vi "1553B-PACKET-2.vi"(0 "数组输入":u8[](array[numeric])) -> (1 "东向加速度":i32, 2 "地向力加速度":i32, 3 "传感器信号":cluster{"陀螺温度":i16, "加计温度":i16}, 4 "俯仰角速率":i16, 6 "北向加速度":i32, 8 "滚转角速率":i16, 10 "航向角速率":i16, 12 "法向过载":i16, 13 "轴向过载":i16, 14 "侧向过载":i16, 15 "地向速度":i32)   [LabVIEW 2012]
uses:
  index-i16.vi
  XX-I16.vi
  index-i32.vi
  XX-I32.vi
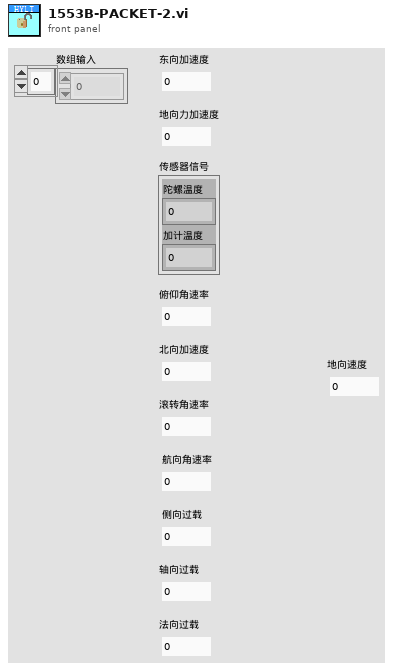
[diagram p1: front panel]
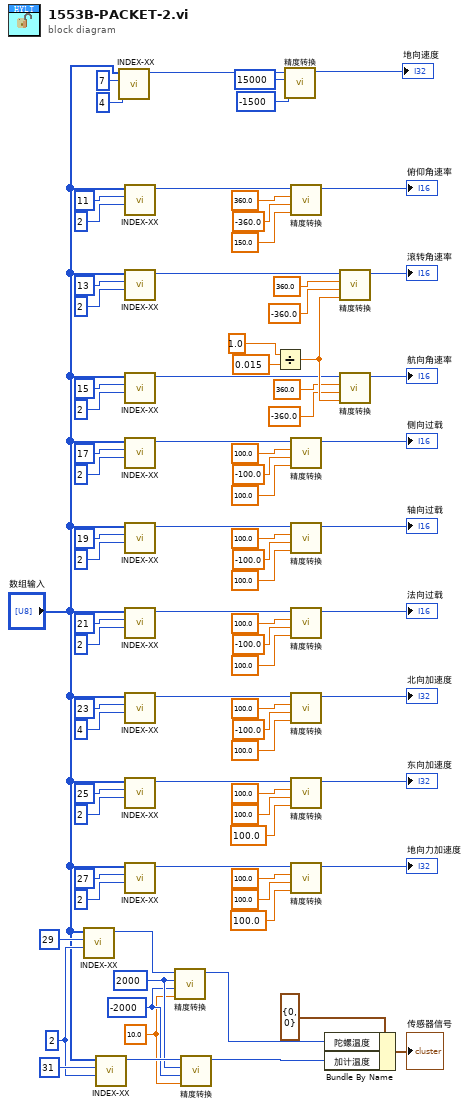
[diagram p0: block diagram]
diagram:
  w11 = i16 -2000 ("下限")
  w12 = i16 2000 ("上限")
  w10 = 10.0 ("单位")
  w13 = 2 ("长度")
  n1 = call-poly "INDEX-XX.vi"("长度"=w13, "索引"=29, "数组"="数组输入") -> ("数值输出"=w16:i16)  [unwired: 8 in]
  n2 = call-poly "INDEX-XX.vi"("长度"=w13, "索引"=31, "数组"="数组输入") -> ("数值输出"=w18:i16)  [unwired: 8 in]
  n3 = call-poly "INDEX-XX.vi"("长度"=4, "索引"=7, "数组"="数组输入") -> ("数值输出"=w2:i32)  [unwired: 8 in]
  n4 = call-poly "INDEX-XX.vi"("长度"=2, "索引"=11, "数组"="数组输入") -> ("数值输出"=w53:i16)  [unwired: 8 in]
  n5 = call-poly "INDEX-XX.vi"("长度"=2, "索引"=13, "数组"="数组输入") -> ("数值输出"=w55:i16)  [unwired: 8 in]
  n6 = call-poly "INDEX-XX.vi"("长度"=2, "索引"=15, "数组"="数组输入") -> ("数值输出"=w58:i16)  [unwired: 8 in]
  n7 = call-poly "INDEX-XX.vi"("长度"=2, "索引"=17, "数组"="数组输入") -> ("数值输出"=w62:i16)  [unwired: 8 in]
  n8 = call-poly "INDEX-XX.vi"("长度"=2, "索引"=19, "数组"="数组输入") -> ("数值输出"=w66:i16)  [unwired: 8 in]
  n9 = call-poly "INDEX-XX.vi"("长度"=2, "索引"=21, "数组"="数组输入") -> ("数值输出"=w70:i16)  [unwired: 8 in]
  n10 = call-poly "INDEX-XX.vi"("长度"=4, "索引"=23, "数组"="数组输入") -> ("数值输出"=w40:i32)  [unwired: 8 in]
  n11 = call-poly "INDEX-XX.vi"("长度"=2, "索引"=25, "数组"="数组输入") -> ("数值输出"=w49:i32)  [unwired: 8 in]
  n12 = call-poly "INDEX-XX.vi"("长度"=2, "索引"=27, "数组"="数组输入") -> ("数值输出"=w20:i32)  [unwired: 8 in]
  n13 = call-poly "精度转换.vi"("单位"=w10, "下限"=w11, "上限"=w12, "数值输入"=w16) -> ("输出"=w17:i16)  [unwired: 7 in]
  n14 = call-poly "精度转换.vi"("单位"=w10, "下限"=w11, "上限"=w12, "数值输入"=w18) -> ("输出"=w19:i16)  [unwired: 7 in]
  n15 = Divide(x=1.0, y=0.015 ("单位")) -> (x/y=w74:dbl)
  n16 = call-poly "精度转换.vi"("下限"=-1500, "上限"=15000, "数值输入"=w2) -> ("输出"=→"地向速度":i32)  [unwired: 8 in]
  n17 = call-poly "精度转换.vi"("单位"=150.0, "下限"=-360.0, "上限"=360.0, "数值输入"=w53) -> ("输出"=→"俯仰角速率":i16)  [unwired: 7 in]
  n18 = call-poly "精度转换.vi"("单位"=100.0, "下限"=-100.0, "上限"=100.0, "数值输入"=w62) -> ("输出"=→"侧向过载":i16)  [unwired: 7 in]
  n19 = call-poly "精度转换.vi"("单位"=100.0, "下限"=-100.0, "上限"=100.0, "数值输入"=w66) -> ("输出"=→"轴向过载":i16)  [unwired: 7 in]
  n20 = call-poly "精度转换.vi"("单位"=100.0, "下限"=-100.0, "上限"=100.0, "数值输入"=w70) -> ("输出"=→"法向过载":i16)  [unwired: 7 in]
  n21 = call-poly "精度转换.vi"("单位"=100.0, "下限"=-100.0, "上限"=100.0, "数值输入"=w40) -> ("输出"=→"北向加速度":i32)  [unwired: 7 in]
  n22 = call-poly "精度转换.vi"("单位"=100.0, "下限"=100.0, "上限"=100.0, "数值输入"=w49) -> ("输出"=→"东向加速度":i32)  [unwired: 7 in]
  n23 = call-poly "精度转换.vi"("单位"=100.0, "下限"=100.0, "上限"=100.0, "数值输入"=w20) -> ("输出"=→"地向力加速度":i32)  [unwired: 7 in]
  n24 = Bundle By Name(cluster=cluster{"陀螺温度":i16, "加计温度":i16} {"陀螺温度"=0, "加计温度"=0} ("传感器信号 3"), "陀螺温度"=w17, "加计温度"=w19) -> (→"传感器信号":cluster{"陀螺温度":i16, "加计温度":i16})
  n25 = call-poly "精度转换.vi"("单位"=w74, "下限"=-360.0, "上限"=360.0, "数值输入"=w55) -> ("输出"=→"滚转角速率":i16)  [unwired: 7 in]
  n26 = call-poly "精度转换.vi"("单位"=w74, "下限"=-360.0, "上限"=360.0, "数值输入"=w58) -> ("输出"=→"航向角速率":i16)  [unwired: 7 in]
